vi "Write Pico Parameter.vi"(8 "error in (no error)":errorcluster, 10 "Pico Parameters":T1={"Pico Type"=enum."Open-Loop Pico", "Acceleration (steps/sec^2)"="20000", "Velocity ( Hz)"="2000", "Driver"="A1", "Motor"="M0", "Channel"="M0", "Process Step"=""}, 11 "PicomotorAxis in":refnum<class "PicomotorController.lvclass">) -> (0 "error out":errorcluster, 3 "PicomotorAxis out":refnum<class "PicomotorController.lvclass">)   [LabVIEW 2020, in "PicomotorController.lvclass"]
uses:
  PicomotorController.lvclass
  subvis/Example_LabVIEW 6.1_MCL Rev E.llb/Pico Parameters.ctl
  PicomotorController.lvclass/PicomotorController.ctl
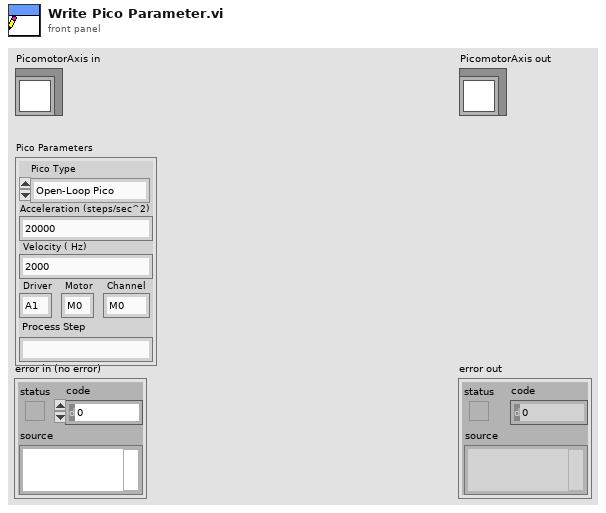
[diagram p1: front panel]
types:
  T1 = typedef "Pico Parameters.ctl" = cluster{"Pico Type":enum16{"Open-Loop Pico", "Close-Loop Pico", "Pico Ultra"}, "Acceleration (steps/sec^2)":string, "Velocity ( Hz)":string, "Driver":string, "Motor":string, "Channel":string, "Process Step":string}
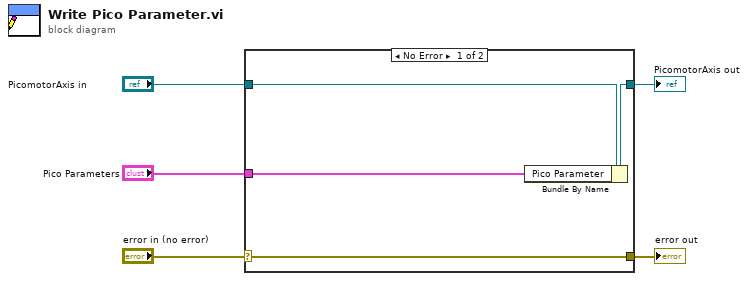
[diagram p0: block diagram]
diagram:
  n1 = case shown="No Error" "error in (no error)" {
    selector: "error in (no error)" -> [w9 w10]
    tunnel: [w9 w10] -> w4
    tunnel: [w7 w11] -> w2
    tunnel: "PicomotorAxis in" -> [w8 w11]
    tunnel: "Pico Parameters" -> [w6 _]
    frame No Error {
      n2 = Bundle By Name(cluster=w8, "Pico Parameter"=w6) -> (w7:refnum<class "PicomotorController.lvclass">)
    }
    frame Error {
    }
  }
  "error out" <- w4
  "PicomotorAxis out" <- w2
